vi "Tester.vi"() -> ()   [LabVIEW 2018]
panel:
  out "refnum out":refnum<file>
  out "error out":errorcluster
  in  "file path (use dialog)":path=path "C:/abc.def"
  in  "error in":errorcluster
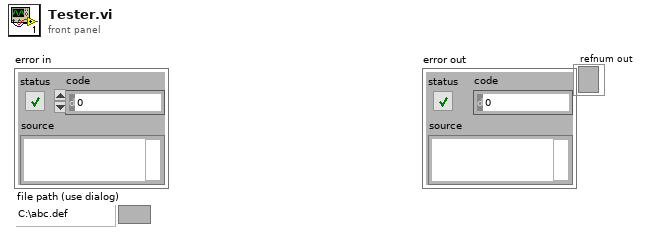
[diagram p1: front panel]
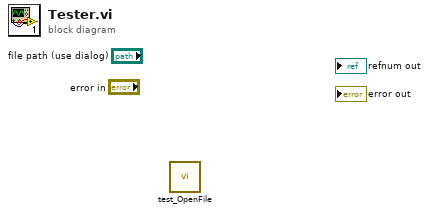
[diagram p0: block diagram]
diagram:
  n1 = call "test_OpenFile.vi"() -> ()  [unwired: 10 in, 2 out]
